vi "Tension Conversion.vi"(8 "error in":errorcluster, 10 "Spoke Type":T1, 11 "Tension Input":dbl) -> (0 "error out":errorcluster, 2 "Out of range":bool, 3 "Tension [kgf]":dbl)   [LabVIEW 2025]
uses:
  Controls/Spork type.ctl
  Controls/Tencion Conversion Table.ctl
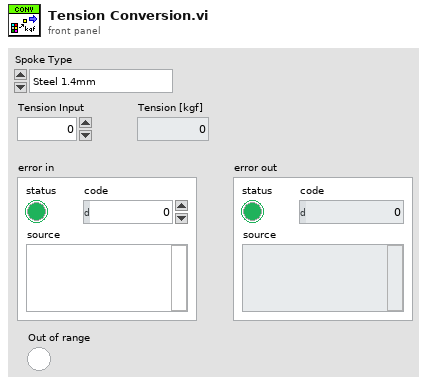
[diagram p1: front panel]
types:
  T1 = typedef "Spork type.ctl" = enum16{"Steel 1.4mm", "Steel 1.5mm", "Steel 1.6mm", "Steel 1.7mm", "Steel 1.8mm", "Steel 2mm", "Steel 2.3mm", "Steel 2.5mm", "Steel 2.6mm", "Aluminum 2.28mm", "Aluminum 2.54mm", "Aluminum 2.8mm", "Aluminum 3.3mm"}
  T2 = typedef "Tencion Conversion Table.ctl" = dbl[][]
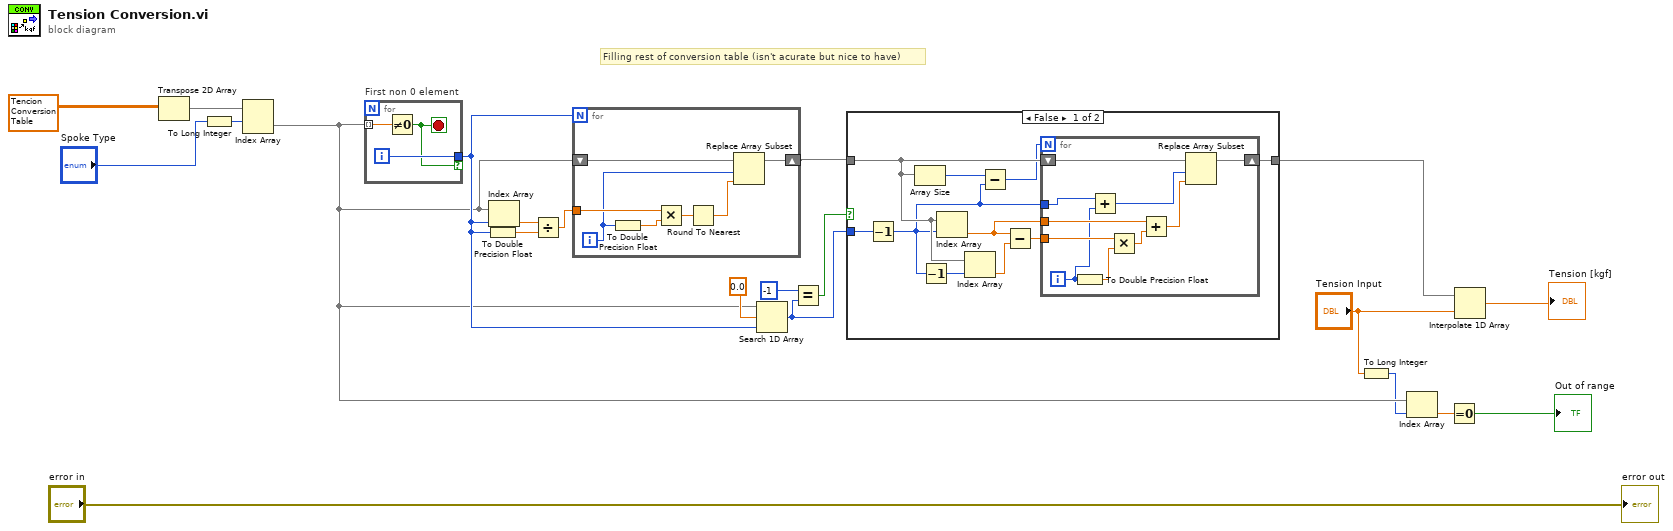
[diagram p0: block diagram]
diagram:
  # "Filling rest of conversion table (isn't acurate but nice to have)"
  n1 = Transpose 2D Array(2D array=T2 [[0.0, 0.0, 0.0, 0.0, 0.0, 0.0, 0.0, 0.0, 0.0, 0.0, 0.0, 0.0, 0.0], [0.0, 0.0, 0.0, 0.0, 0.0, 0.0, 0.0, 0.0, 0.0, 0.0, 0.0, 0.0, 0.0], [0.0, 0.0, 0.0, 0.0, 0.0, 0.0, 0.0, 0.0, 0.0, 0.0, 0.0, 0.0, 0.0], [0.0, 0.0, 0.0, 0.0, 0.0, 0.0, 0.0, 0.0, 0.0, 0.0, 0.0, 0.0, 0.0], [0.0, 0.0, 0.0, 0.0, 0.0, 0.0, 0.0, 0.0, 0.0, 0.0, 0.0, 0.0, 0.0], [0.0, 0.0, 0.0, 0.0, 0.0, 0.0, 0.0, 0.0, 0.0, 0.0, 0.0, 0.0, 0.0], [0.0, 0.0, 0.0, 0.0, 0.0, 0.0, 0.0, 0.0, 0.0, 0.0, 0.0, 0.0, 0.0], [0.0, 0.0, 0.0, 0.0, 0.0, 0.0, 0.0, 0.0, 0.0, 0.0, 0.0, 0.0, 0.0], [54.0, 0.0, 0.0, 0.0, 0.0, 0.0, 0.0, 0.0, 0.0, 0.0, 0.0, 0.0, 0.0], [58.0, 52.0, 0.0, 0.0, 0.0, 0.0, 0.0, 0.0, 0.0, 0.0, 0.0, 0.0, 0.0], [63.0, 56.0, 0.0, 0.0, 0.0, 0.0, 0.0, 0.0, 0.0, 0.0, 0.0, 0.0, 0.0], [69.0, 61.0, 54.0, 0.0, 0.0, 0.0, 0.0, 0.0, 0.0, 0.0, 0.0, 0.0, 0.0], [75.0, 66.0, 58.0, 51.0, 0.0, 0.0, 0.0, 0.0, 0.0, 0.0, 0.0, 0.0, 0.0], [83.0, 73.0, 64.0, 56.0, 0.0, 0.0, 0.0, 0.0, 0.0, 0.0, 0.0, 0.0, 0.0], [91.0, 80.0, 70.0, 61.0, 53.0, 0.0, 0.0, 0.0, 0.0, 0.0, 0.0, 0.0, 0.0], [100.0, 88.0, 76.0, 67.0, 58.0, 0.0, 0.0, 0.0, 0.0, 52.0, 0.0, 0.0, 0.0], [111.0, 97.0, 84.0, 73.0, 64.0, 0.0, 0.0, 0.0, 0.0, 55.0, 0.0, 0.0, 0.0], [123.0, 107.0, 93.0, 81.0, 70.0, 53.0, 0.0, 0.0, 0.0, 59.0, 0.0, 0.0, 0.0], [137.0, 119.0, 103.0, 89.0, 77.0, 58.0, 0.0, 0.0, 0.0, 64.0, 0.0, 0.0, 0.0], [154.0, 133.0, 114.0, 99.0, 85.0, 63.0, 0.0, 0.0, 0.0, 69.0, 0.0, 0.0, 0.0], [172.0, 148.0, 128.0, 110.0, 94.0, 70.0, 0.0, 0.0, 0.0, 74.0, 52.0, 0.0, 0.0], [0.0, 166.0, 143.0, 122.0, 105.0, 77.0, 0.0, 0.0, 0.0, 80.0, 57.0, 0.0, 0.0], [0.0, 0.0, 160.0, 137.0, 117.0, 86.0, 54.0, 0.0, 0.0, 87.0, 62.0, 0.0, 0.0], [0.0, 0.0, 0.0, 154.0, 131.0, 96.0, 59.0, 0.0, 0.0, 94.0, 68.0, 0.0, 0.0], [0.0, 0.0, 0.0, 174.0, 148.0, 107.0, 66.0, 0.0, 0.0, 102.0, 75.0, 0.0, 0.0], [0.0, 0.0, 0.0, 0.0, 167.0, 120.0, 73.0, 53.0, 0.0, 111.0, 82.0, 51.0, 0.0], [0.0, 0.0, 0.0, 0.0, 0.0, 135.0, 82.0, 59.0, 0.0, 122.0, 91.0, 57.0, 0.0], [0.0, 0.0, 0.0, 0.0, 0.0, 153.0, 92.0, 66.0, 55.0, 133.0, 100.0, 63.0, 0.0], [0.0, 0.0, 0.0, 0.0, 0.0, 173.0, 104.0, 73.0, 62.0, 146.0, 110.0, 70.0, 0.0], [0.0, 0.0, 0.0, 0.0, 0.0, 0.0, 117.0, 83.0, 69.0, 160.0, 122.0, 79.0, 0.0], [0.0, 0.0, 0.0, 0.0, 0.0, 0.0, 133.0, 93.0, 78.0, 176.0, 135.0, 88.0, 0.0], [0.0, 0.0, 0.0, 0.0, 0.0, 0.0, 151.0, 106.0, 88.0, 0.0, 150.0, 98.0, 0.0], [0.0, 0.0, 0.0, 0.0, 0.0, 0.0, 172.0, 120.0, 100.0, 0.0, 167.0, 110.0, 0.0], [0.0, 0.0, 0.0, 0.0, 0.0, 0.0, 0.0, 137.0, 114.0, 0.0, 0.0, 124.0, 56.0], [0.0, 0.0, 0.0, 0.0, 0.0, 0.0, 0.0, 157.0, 130.0, 0.0, 0.0, 140.0, 65.0], [0.0, 0.0, 0.0, 0.0, 0.0, 0.0, 0.0, 0.0, 150.0, 0.0, 0.0, 157.0, 76.0], [0.0, 0.0, 0.0, 0.0, 0.0, 0.0, 0.0, 0.0, 172.0, 0.0, 0.0, 178.0, 89.0], [0.0, 0.0, 0.0, 0.0, 0.0, 0.0, 0.0, 0.0, 0.0, 0.0, 0.0, 0.0, 105.0], [0.0, 0.0, 0.0, 0.0, 0.0, 0.0, 0.0, 0.0, 0.0, 0.0, 0.0, 0.0, 123.0], [0.0, 0.0, 0.0, 0.0, 0.0, 0.0, 0.0, 0.0, 0.0, 0.0, 0.0, 0.0, 146.0], [0.0, 0.0, 0.0, 0.0, 0.0, 0.0, 0.0, 0.0, 0.0, 0.0, 0.0, 0.0, 174.0]] ("Tencion Conversion Table")) -> (transposed array=w12:T2)
  n2 = To Long Integer(number="Spoke Type") -> (32bit integer=w7:i32)
  n3 = Index Array(array=w12, index (row)=w7) -> (element=w5:dbl[])  [unwired: 1 in]
  n4 = for "First non 0 element" {
    tunnel: w5 -> [w24] mode=indexing
    tunnel: [w23] -> w18 if=w22
    i -> [w23]
    stop <- w22 stop-if-true
    n5 = Not Equal To 0?(x=w24) -> (x != 0?=w22:bool)
  }
  n6 = To Double Precision Float(number=w18) -> (double precision float=w20:dbl)
  n7 = Index Array(array=w5, index=w18) -> (element=w21:dbl)
  n8 = Divide(x=w21, y=w20) -> (x/y=w19:dbl)
  n9 = for {
    N: w18 -> [_]
    tunnel: w19 -> [w30]
    shift-right: [w27] -> w16
    shift-left: w5 -> [w31]
    i -> [w28]
    n10 = To Double Precision Float(number=w28) -> (double precision float=w29:dbl)
    n11 = Multiply(x=w30, y=w29) -> (x*y=w26:dbl)
    n12 = Round To Nearest(number=w26) -> (nearest integer value=w25:dbl)
    n13 = Replace Array Subset(array=w31, new element=w25, index=w28) -> (w27:dbl[])
  }
  n14 = Search 1D Array(1D array=w5, element=0.0, start index (0)=w18) -> (index of element=w13:i32)
  n15 = Equal?(x=-1, y=w13) -> (x = y?=w14:bool)
  n16 = case shown="False" w14 {
    tunnel: [w35 w52] -> w10
    tunnel: w16 -> [w37 w52]
    tunnel: w13 -> [w34 _]
    frame False {
      n17 = Decrement(x=w34) -> (x-1=w32:i32)
      n18 = Array Size(array=w37) -> (size(s)=w39:i32)
      n19 = Decrement(x=w32) -> (x-1=w41:i32)
      n20 = Index Array(array=w37, index=w32) -> (element=w36:dbl)
      n21 = Index Array(array=w37, index=w41) -> (element=w40:dbl)
      n22 = Subtract(x=w39, y=w32) -> (x-y=w33:i32)
      n23 = Subtract(x=w36, y=w40) -> (x-y=w38:dbl)
      n24 = for {
        N: w33 -> [_]
        tunnel: w38 -> [w50]
        tunnel: w36 -> [w47]
        shift-right: [w45] -> w35
        shift-left: w37 -> [w51]
        tunnel: w32 -> [w42]
        i -> [w44]
        n25 = To Double Precision Float(number=w44) -> (double precision float=w49:dbl)
        n26 = Add(x=w42, y=w44) -> (x+y=w43:i32)
        n27 = Multiply(x=w50, y=w49) -> (x*y=w48:dbl)
        n28 = Add(x=w47, y=w48) -> (x+y=w46:dbl)
        n29 = Replace Array Subset(array=w51, new element=w46, index=w43) -> (w45:dbl[])
      }
    }
    frame True {
    }
  }
  n30 = To Long Integer(number="Tension Input") -> (32bit integer=w4:i32)
  n31 = Index Array(array=w5, index=w4) -> (element=w2:dbl)
  n32 = Equal To 0?(x=w2) -> (x = 0?=→"Out of range":bool)
  n33 = Interpolate 1D Array(1:"Tension Input", 2:w10) -> (0:→"Tension [kgf]":dbl)
  "error out" <- "error in"
